vi "FTW-Event-Construct.vi"(0 "Event Type":string, 5 "Event Data":string, 7 "Source":string="CallChain", 11 "Error to Log":errorcluster) -> (4 "Event":T1 {"Timestamp" format="%<%Y-%m-%d %H:%M:%S%03u>T"; "Uptime" format="%.3ps"})   [LabVIEW 2015]
uses:
  FTW-Event.ctl
panel:
  # "Inputs"
  # "Outputs"
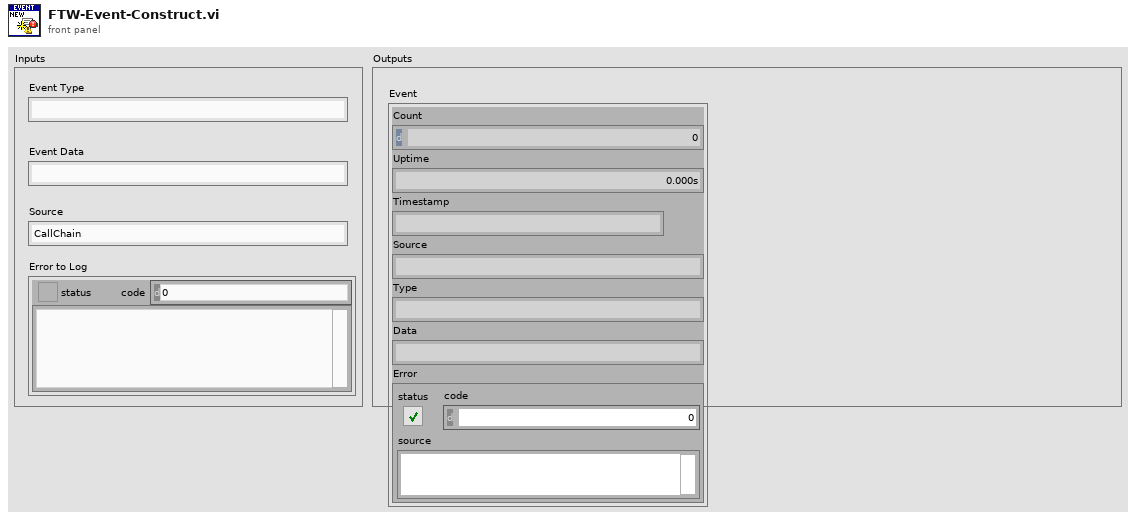
[diagram p1: front panel]
types:
  T1 = typedef "FTW-Event.ctl" = cluster{"Count":i32, "Uptime":dbl, "Timestamp":timestamp, "Source":string, "Type":string, "Data":string, "Error":errorcluster}
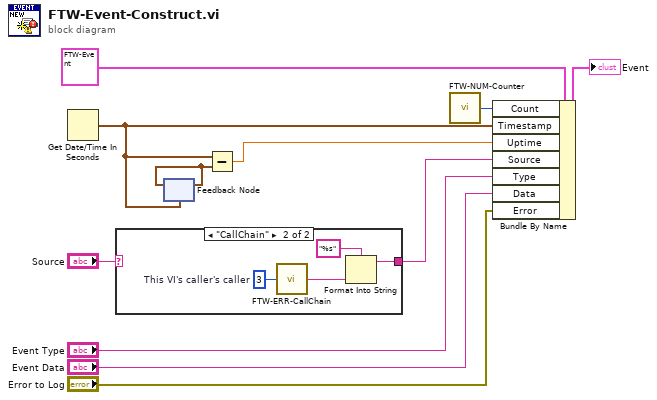
[diagram p0: block diagram]
diagram:
  n1 = Get Date/Time In Seconds() -> (seconds since 1Jan1904=w3:timestamp)
  n2 = case shown="\"CallChain\"" "Source" {
    selector: "Source" -> [w12 _]
    tunnel: [w12 w15] -> w1
    frame Default {
    }
    frame "CallChain" {
      w14 = 3  # This VI's caller's caller
      n3 = call "FTW-ERR-CallChain.vi"("Levels to exclude (1=This VI's caller)"=w14) -> ("Call Chain"=w13:string)
      n4 = Format Into String(format string="%s", w13) -> (resulting string=w15:string)  [unwired: 2 in, 1 out]
    }
  }
  n5 = feedback #1(w3) -> (w9:timestamp)
  n6 = feedback-in #1(w9) -> ()
  n7 = Subtract(x=w3, y=w9) -> (x-y=w4:dbl)
  n8 = call "FTW-NUM-Counter.vi"() -> ("Counter"=w7:i32)  [unwired: 1 in]
  n9 = Bundle By Name(cluster=T1 {"Count"=0, "Uptime"=0.0, "Timestamp"=timestamp(0 s since 1904-01-01), "Source"="", "Type"="", "Data"="", "Error"={"status"=FALSE, "code"=0, "source"=""}} ("Event"), "Count"=w7, "Timestamp"=w3, "Uptime"=w4, "Source"=w1, "Type"="Event Type", "Data"="Event Data", "Error"="Error to Log") -> (→"Event":T1)
